vi "Configure SOS 0.vi"(8 "error in (no error)":errorcluster, 10 "lock-in.iir config 0":T1 {"b0" format="%.17g"; "b1" format="%.17g"; "-a1" format="%.17g"; "-a2" format="%.17g"}, 11 "LIA Host Interface in":refnum<class "LIA Host Interface.lvclass">) -> (0 "error out":errorcluster, 3 "LIA Host Interface out":refnum<class "LIA Host Interface.lvclass">)   [LabVIEW 2017, in "LIA Debugging.lvclass"]
uses:
  LIA Debugging.lvclass
  Program Files (x86)/National Instruments/LabVIEW 2017/examples/Lock-In Amplifier/lib/interface/Interface/LIA Host Interface.lvclass
  Program Files (x86)/National Instruments/LabVIEW 2017/examples/Lock-In Amplifier/lib/interface/Interface FPGA/LIA Host Interface FPGA.lvclass
  Program Files (x86)/National Instruments/LabVIEW 2017/examples/Lock-In Amplifier/lib/interface/Interface FPGA/Properties/FpgaSession_GET.vi
  <vilib>/Utility/error.llb/Error Cluster From Error Code.vi
  <vilib>/rvi/errors/niLvFpgaAdjustHostInterfaceError.vi
  <vilib>/rvi/interface/nirviReadWriteControl/nirviReadWriteControl.xnode
  <vilib>/rvi/interface/Simulation/niFpgaSimulationCallBeginRW.vi
  NiFpgaLv.dll
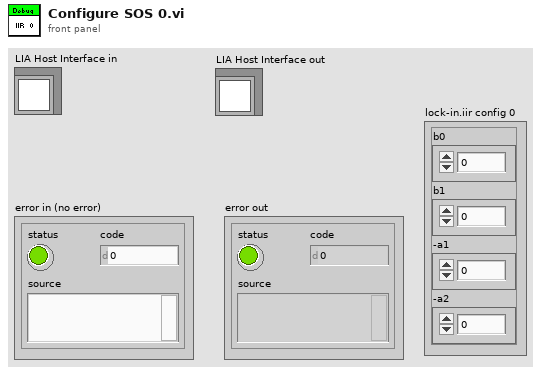
[diagram p1: front panel]
types:
  T1 = cluster{"b0":fxp<+/-,18,2>, "b1":fxp<+/-,18,2>, "-a1":fxp<+/-,18,2>, "-a2":fxp<+/-,18,2>}
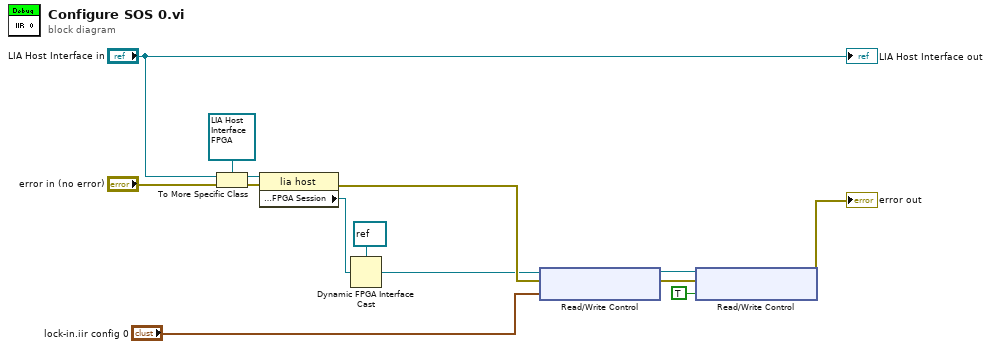
[diagram p0: block diagram]
diagram:
  n1 = To More Specific Class(target class=refnum<class "LIA Host Interface FPGA.lvclass"> refnum ("lia host"), reference="LIA Host Interface in", error in="error in (no error)") -> (specific class reference=w9:refnum<class "LIA Host Interface FPGA.lvclass">, error out=w8:errorcluster)
  n2 = property class="lia host"(reference=w9, error in=w8) -> (error out=w13:errorcluster, "Properties:FPGA Session"=w5:refnum<k20>)  [unwired: 1 out]
  n3 = Dynamic FPGA Interface Cast(Session In=refnum<k20> refnum ("fpga type"), Type=w5) -> (Session Out=w7:refnum<k20>)
  n4 = xnode "Read/Write Control"("FPGA VI Reference In"=w7, "error in"=w13, "lock-in.iir config0 0"="lock-in.iir config 0") -> ("FPGA VI Reference Out"=w10:refnum<k20>, "error out"=w11:errorcluster)
  n5 = xnode "Read/Write Control"("FPGA VI Reference In"=w10, "error in"=w11, "lock-in.iir enable0 0"=TRUE ("nco.reset 0")) -> ("error out"=→"error out":errorcluster)  [unwired: 1 out]
  "LIA Host Interface out" <- "LIA Host Interface in"
